vi "ZeroMQ Client.vi"() -> ()   [LabVIEW 2018]
uses:
  <vilib>/addons/zeromq/socket_type.ctl
  <vilib>/addons/zeromq/zmq_socket.lvclass
  <vilib>/addons/zeromq/zmq_context.lvclass
  <vilib>/addons/zeromq/zeromq.lvlib
panel:
  in  "stop":bool
  in  "command":string="S4ICS"
  in  "endpoint":string="tcp://127.0.0.1:5555"
  out "status":string
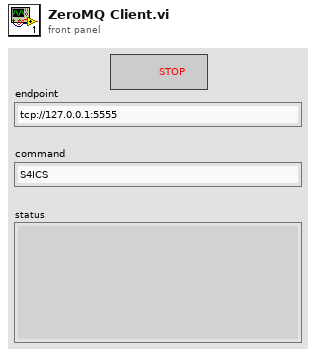
[diagram p1: front panel]
types:
  T1 = typedef "zeromq.lvlib/socket_type.ctl" = enum8{"ZMQ_PAIR", "ZMQ_PUB", "ZMQ_SUB", "ZMQ_REQ", "ZMQ_REP", "ZMQ_DEALER", "ZMQ_ROUTER", "ZMQ_PULL", "ZMQ_PUSH", "ZMQ_XPUB", "ZMQ_XSUB", "ZMQ_STREAM", "ZMQ_SERVER", "ZMQ_CLIENT", "ZMQ_RADIO", "ZMQ_DISH", "ZMQ_GATHER", "ZMQ_SCATTER", "ZMQ_DGRAM"}
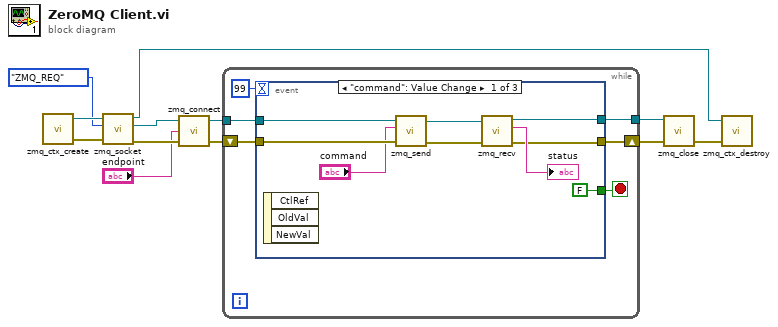
[diagram p0: block diagram]
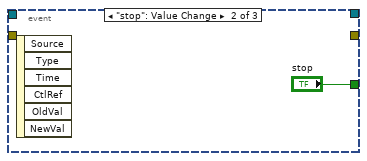
[diagram p2: hidden frame]
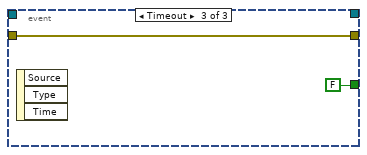
[diagram p3: hidden frame]
diagram:
  n1 = call <vilib>:"zmq_ctx_create.vi"() -> ("error out"=w11:errorcluster, "context out"=w12:refnum<class "zmq_context.lvclass">)  [unwired: 4 in]
  n2 = call <vilib>:"zmq_socket.vi"("error in"=w11, "socket type"=socket_type."ZMQ_REQ", "context in"=w12) -> ("error out"=w9:errorcluster, "socket out"=w6:refnum<class "zmq_socket.lvclass">, "context out"=w10:refnum<class "zmq_context.lvclass">)  [unwired: 2 in]
  n3 = call <vilib>:"zmq_connect.vi"("error in"=w9, "endpoint"="endpoint", "socket in"=w6) -> ("error out"=w7:errorcluster, "socket out"=w8:refnum<class "zmq_socket.lvclass">)  [unwired: 1 in]
  n4 = while {
    tunnel: w8 -> [w18]
    shift-right: [w17] -> w3
    shift-left: w7 -> [w16]
    tunnel: [w13] -> w2
    stop <- w15 stop-if-true
    n5 = event shown="[0] \"command\": Value Change" {
      selector: _ -> [_ _ _]
      dyn-events: _ -> [_ _ _]
      timeout: 99 -> [_ _ _]
      tunnel: w18 -> [w27 _ _]
      tunnel: [w20 _ w30] -> w17
      tunnel: w16 -> [w24 _ w30]
      tunnel: [FALSE "stop" FALSE] -> w15
      tunnel: [w19 _ _] -> w13
      event "command": Value Change {
        n6 = event-data() -> ()  [unwired: 1 in, 3 out]
        n7 = call <vilib>:"zmq_send.vi"("error in"=w24, "data"="command", "socket in"=w27) -> ("error out"=w25:errorcluster, "socket out"=w26:refnum<class "zmq_socket.lvclass">)  [unwired: 4 in]
        n8 = call <vilib>:"zmq_recv.vi"("error in"=w25, "socket in"=w26) -> ("error out"=w20:errorcluster, "data"=→"status":string, "socket out"=w19:refnum<class "zmq_socket.lvclass">)  [unwired: 3 in, 2 out]
      }
      event "stop": Value Change {
        n9 = event-data() -> ()  [unwired: 1 in, 6 out]
      }
      event Timeout {
        n10 = event-data() -> ()  [unwired: 1 in, 3 out]
      }
    }
  }
  n11 = call <vilib>:"zmq_close.vi"("error in"=w3, "socket"=w2) -> ("error out"=w1:errorcluster)  [unwired: 3 in]
  n12 = call <vilib>:"zmq_ctx_destroy.vi"("error in"=w1, "context in"=w10) -> ()  [unwired: 3 in, 1 out]
